vi "Check Solution.vi"() -> ()   [LabVIEW 2013]
uses:
  Classes/GA_Class/Controls/GanntChart_Element.ctl
  Classes/OSSP_Problem.lvclass
  Classes/GA_Class/GA_Operation_To_MachineJobTuple.vi
  Classes/GA_Class/Find Gaps On Particular Machine.vi
  Classes/GA_Class/GA_Check_Other_Machines.vi
  Classes/GA_Class/GA_Schedule_Job.vi
  Classes/GA_Class/GA_Find_Job_On_Other_Machines.vi
  Classes/GA_Class/GA_Increment_NumberofJobsOn Machine_ByOne.vi
  Classes/GA.lvclass
panel:
  out "Processing Times":u16[][](array[numeric])
  out "Gannt Chart Out":T1[][](array[typedef])
  in  "Schedule 1":i32[](array[numeric])
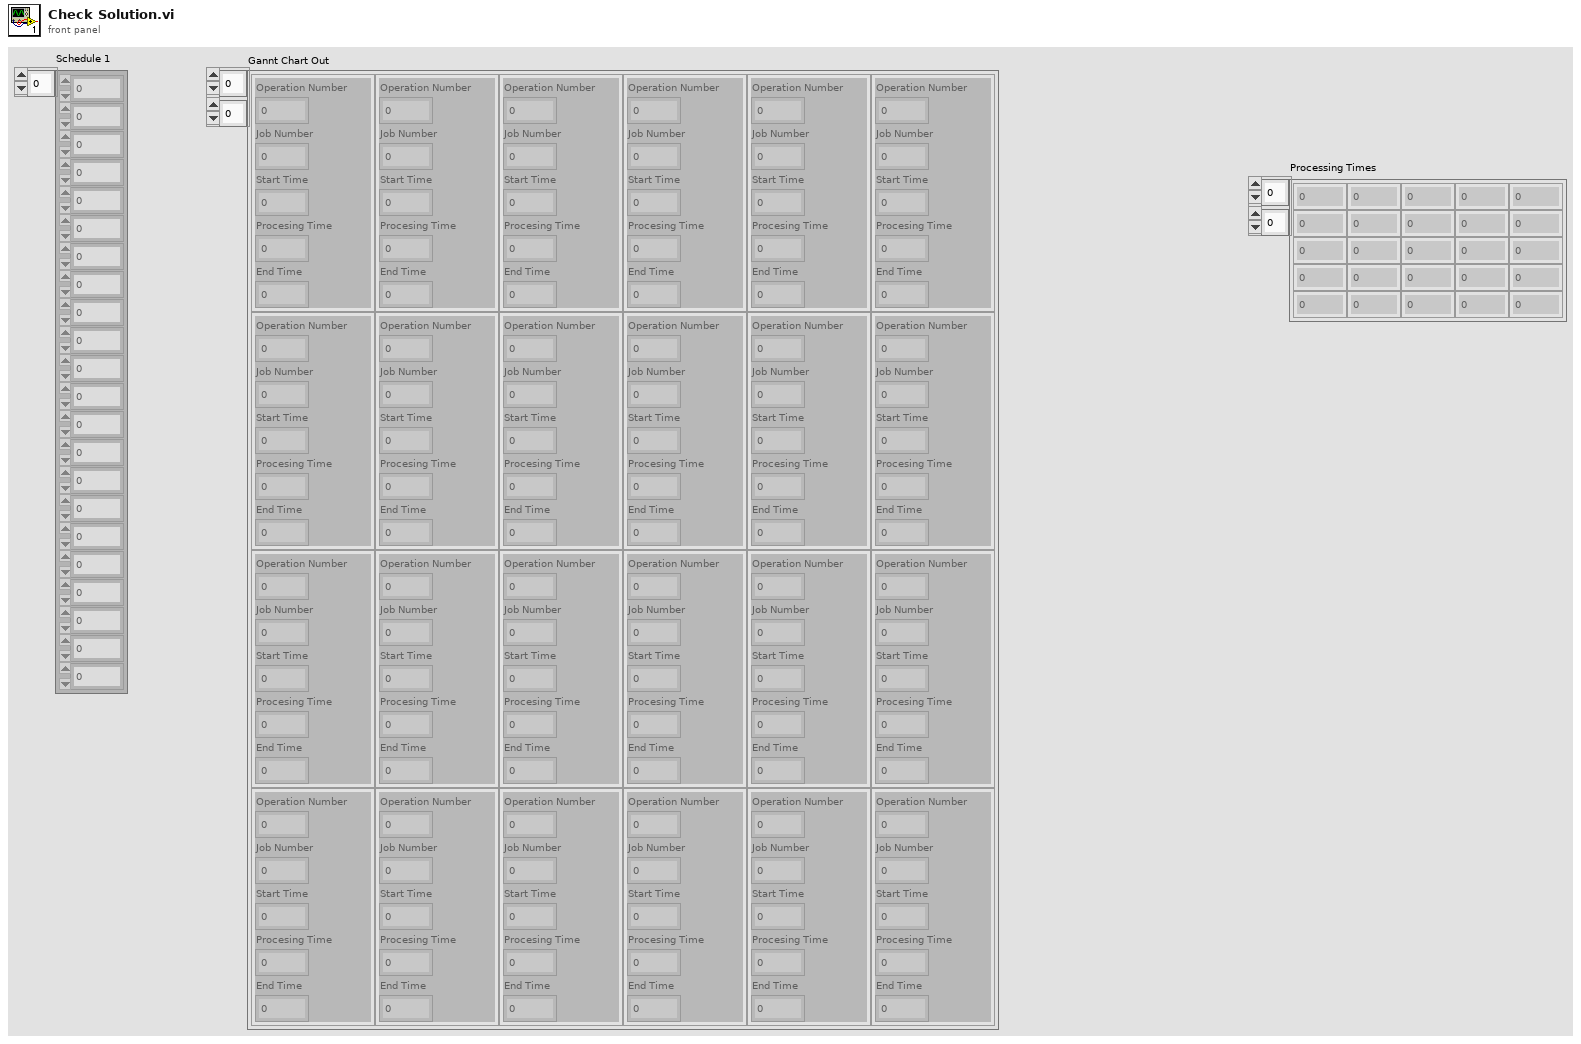
[diagram p1: front panel]
types:
  T1 = typedef "GanntChart_Element.ctl" = cluster{"Operation Number":i32, "Job Number":i32, "Start Time":i32, "Procesing Time":u16, "End Time":i32}
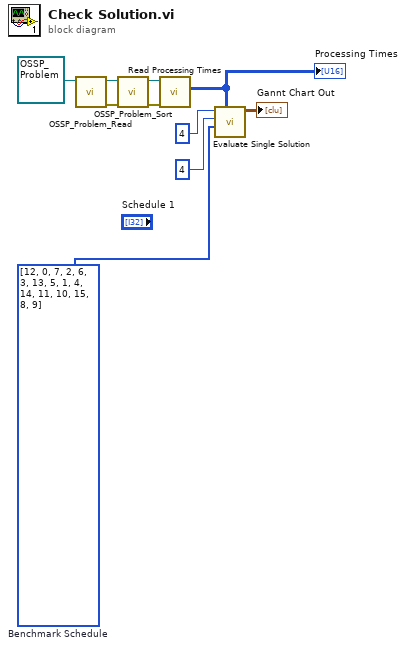
[diagram p0: block diagram]
diagram:
  w1 = i32[] [12, 0, 7, 2, 6, 3, 13, 5, 1, 4, 14, 11, 10, 15, 8, 9]  # Benchmark Schedule
  n1 = call "OSSP_Problem_Read.vi"("OSSP_Problem.lvclass In"=refnum<class "OSSP_Problem.lvclass"> refnum ("OSSP_Problem.lvclass")) -> ("error out"=w8:errorcluster, "OSSP_Problem.lvclass Out"=w9:refnum<class "OSSP_Problem.lvclass">)  [unwired: 9 in]
  n2 = call "OSSP_Problem_Sort.vi"("error in (no error)"=w8, "OSSP_Problem.lvclass In"=w9) -> ("error out"=w6:errorcluster, "OSSP_Problem.lvclass Out"=w7:refnum<class "OSSP_Problem.lvclass">)  [unwired: 8 in]
  n3 = call-dynamic "Read Processing Times.vi"("error in (no error)"=w6, "OSSP_Problem in"=w7) -> ("Processing Times"=w5:u16[][])  [unwired: 7 in, 2 out]
  "Processing Times" <- w5
  n4 = call "Evaluate Single Solution.vi"("Processing Times (Rows Mach.Cols Jobs)"=w5, "Schedule"=w1, "Number of Jobs"=4, "Number of Machines"=4 ("Number of Jobs")) -> ("Gannt Chart Out"=→"Gannt Chart Out":T1[][])  [unwired: 7 in]
